vi "test_RT driver Mockup.vi"() -> ()   [LabVIEW 2020]
uses:
  <instrlib>/BTI1553Lib/Public/Controls/1553 RT Transfer Type.ctl
  <instrlib>/BTI1553Lib/Public/Controls/1553 Transfer Direction.ctl
  _typedefs/rtdm_states_type.ctl
  <instrlib>/BTICardLib/Public/Controls/1553 Record.ctl
  _typedefs/rtdm_reference_types.ctl
  <extravilib>/ChannelInstances/Tag-bool/Write With Abort.vi
  <extravilib>/ChannelInstances/Tag-bool/Read With Abort.vi
  <instrlib>/BTICardLib/Private/Initialize By Card Number and Core Number.vi
  <instrlib>/BTI1553Lib/Private/Channel/Configure/Configure All From XML.vi
  <instrlib>/BTI1553Lib/Private/RT/Configure/Get RT Xfer Handle.vi
  <extravilib>/ChannelInstances/Tag-bool/Instantiate.vi
  <extravilib>/ChannelInstances/Tag-bool/Endpoint.vi
  <extravilib>/ChannelInstances/Tag-bool/EndpointRead.vi
  <instrlib>/BTICardLib/BTICardLV.lvlib
  <instrlib>/BTI1553Lib/BTI1553LV.lvlib
  <extravilib>/ChannelInstances/Tag-bool.lvlib
panel:
  out "data word count out":i32
  out "error out async":errorcluster
  out "error out inline":errorcluster
  in  "Stop operating":bool
  in  "Async period ms":u32=10
  in  "data words":u16[](array[numeric]) format="%04x"
  in  "message type":enum16{"BC-RT", "RT-BC_RT"}(ring)
  out "byte count":i32
  out "last record":T1 {"type" format="%04x"; "activity" format="%04x"; "error" format="%04x"; "cwd1" format="%04x"; "cwd2" format="%04x"; "swd1" format="%04x"; "swd2" format="%04x"; "data" format="%04x"}
  in  "inline period mS":u32=10
  out "current state":T2=enum."Close"
  in  "transfer sa number or mc number":i32=2
  in  "transfer direction":T3 items=["DIRECTION_RECEIVE", "DIRECTION_TRANSMIT"]
  in  "transfer type":T4 items=["RTXFER_SUBADDRESS", "RTXFER_MODECODE"]
  in  "rt address":i32=1
  in  "rt channel":i32
  in  "bc command name":string="testTransfer"
  in  "bc channel index":i32
  out "Product String":string="222-555-442"
  out "Card Type":string="OmniBus II cPCIe/PXIe"
  out "channel count out":i32=1
  in  "number of channels":i32=1
  out "XML load time ms":u32=10008
  in  "card number":i32=1
  in  "core number":i32
  in  "configuration file path":path=path "c:/ni-rt/VeriStand/Custom Devices/Ballard - 1553/Board_1__Core_0__.xml"
  out "error out":errorcluster
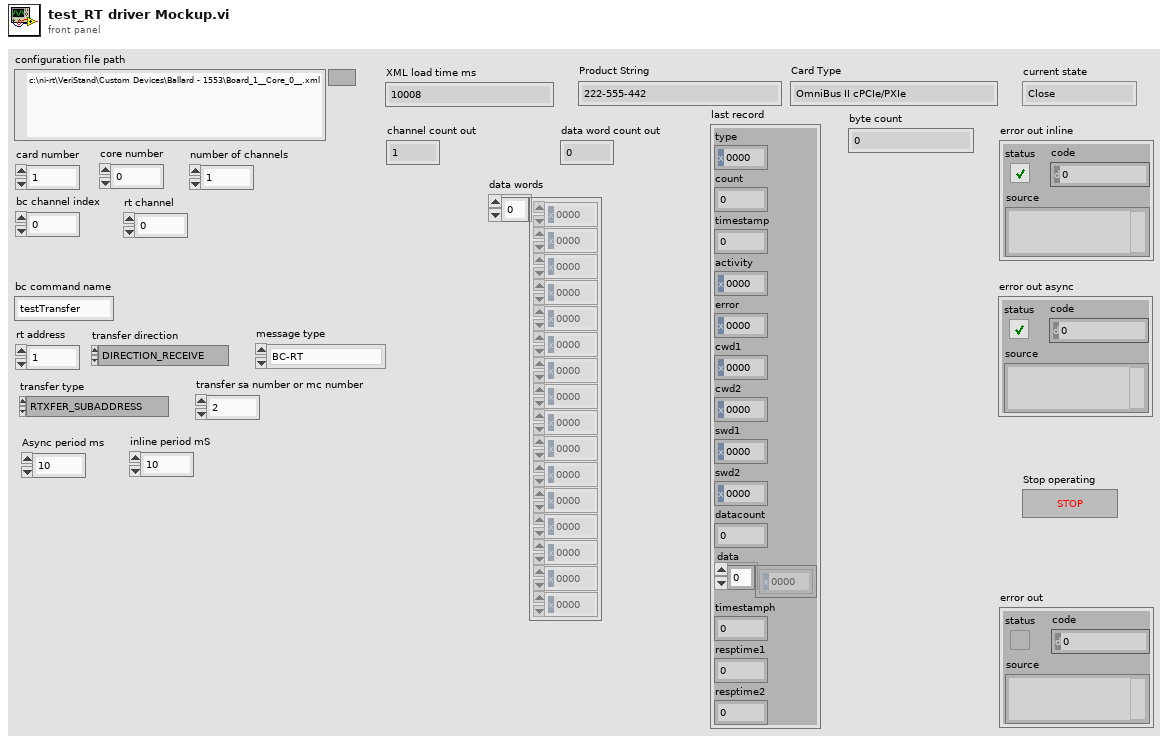
[diagram p1: front panel]
types:
  T1 = typedef "BTICardLV.lvlib/1553 Record.ctl" = cluster{"type":u16, "count":u16, "timestamp":u32, "activity":u16, "error":u16, "cwd1":u16, "cwd2":u16, "swd1":u16, "swd2":u16, "datacount":u16, "data":u16[], "timestamph":u32, "resptime1":u16, "resptime2":u16}
  T2 = typedef "rtdm_states_type.ctl" = enum16{"Initialize", "Get transfer handles", "Operate", "Error", "Close"}
  T3 = typedef "BTI1553LV.lvlib/1553 Transfer Direction.ctl" = u32
  T4 = typedef "BTI1553LV.lvlib/1553 RT Transfer Type.ctl" = u32
  T5 = typedef "rtdm_reference_types.ctl" = cluster{"core handle":u64, "channel handles":u64[], "core reader handle":u64, "bc handle":u64, "bc transfer handle":u64, "rt handle":u64, "rt transfer handle":u64}
  T6 = typedef "Tag-bool.lvlib/))Channel.ctl" = refnum<queue>
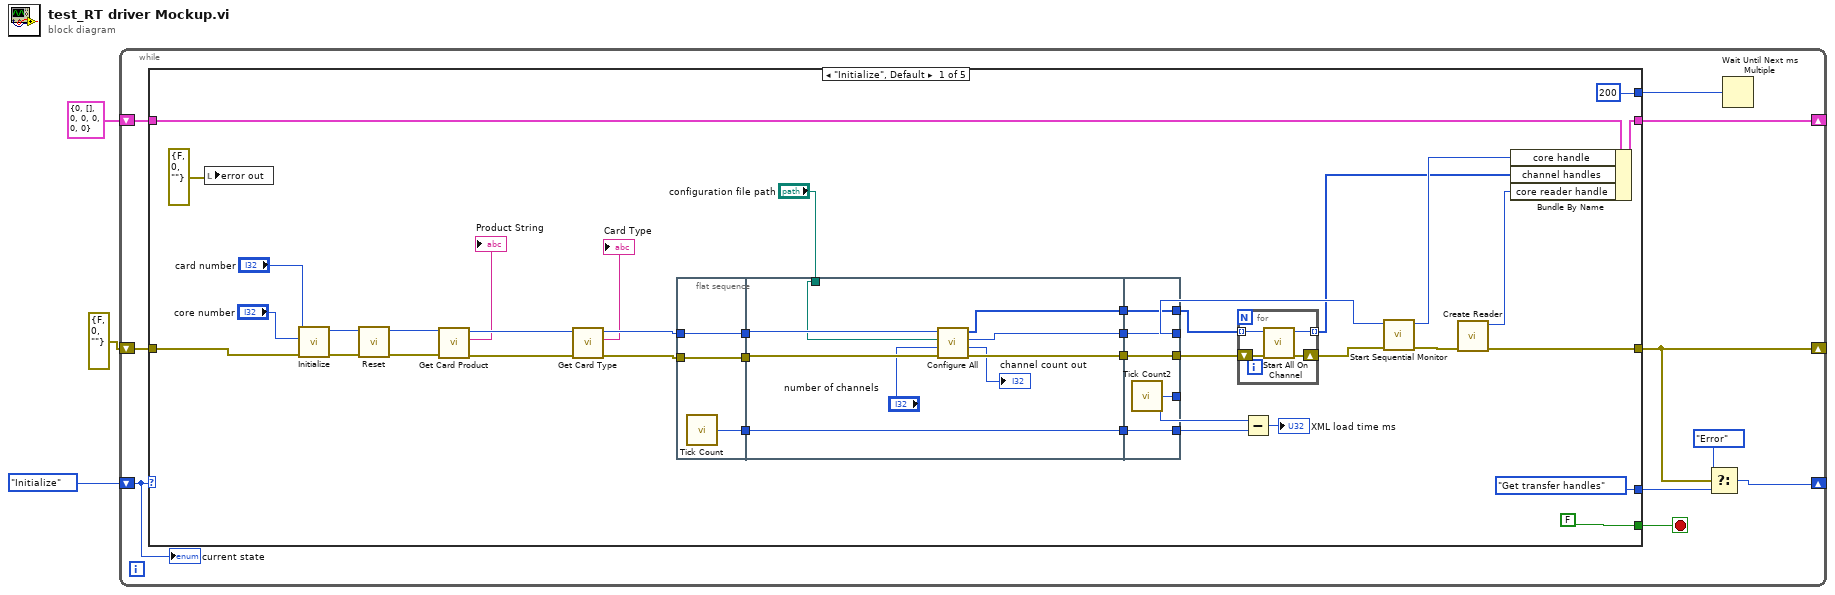
[diagram p0: block diagram]
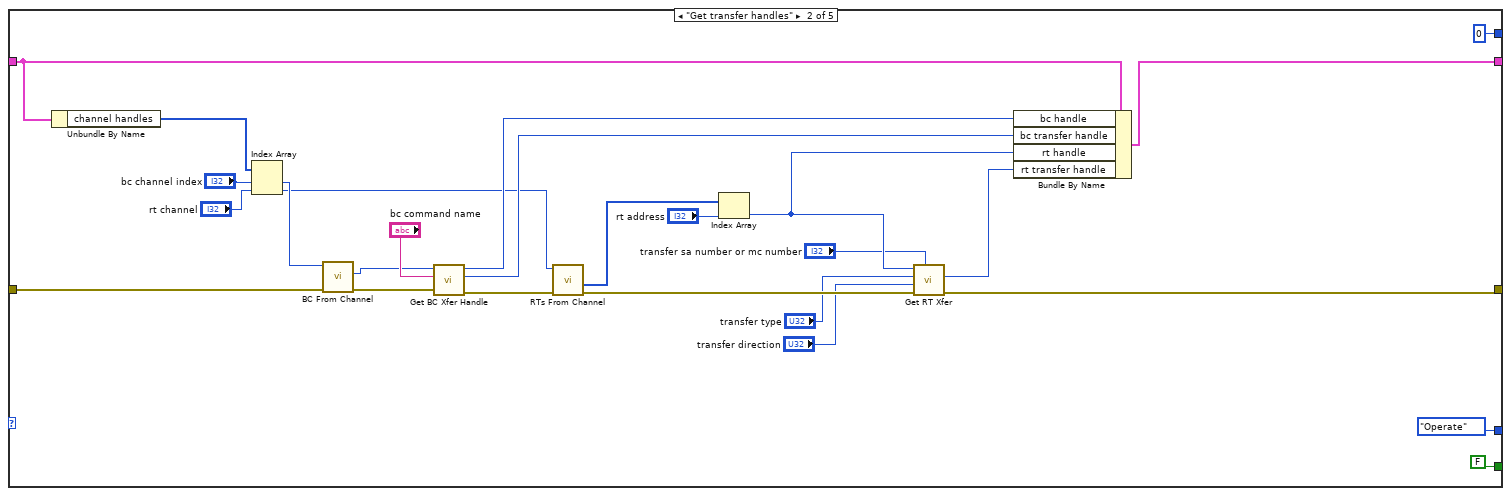
[diagram p2: hidden frame]
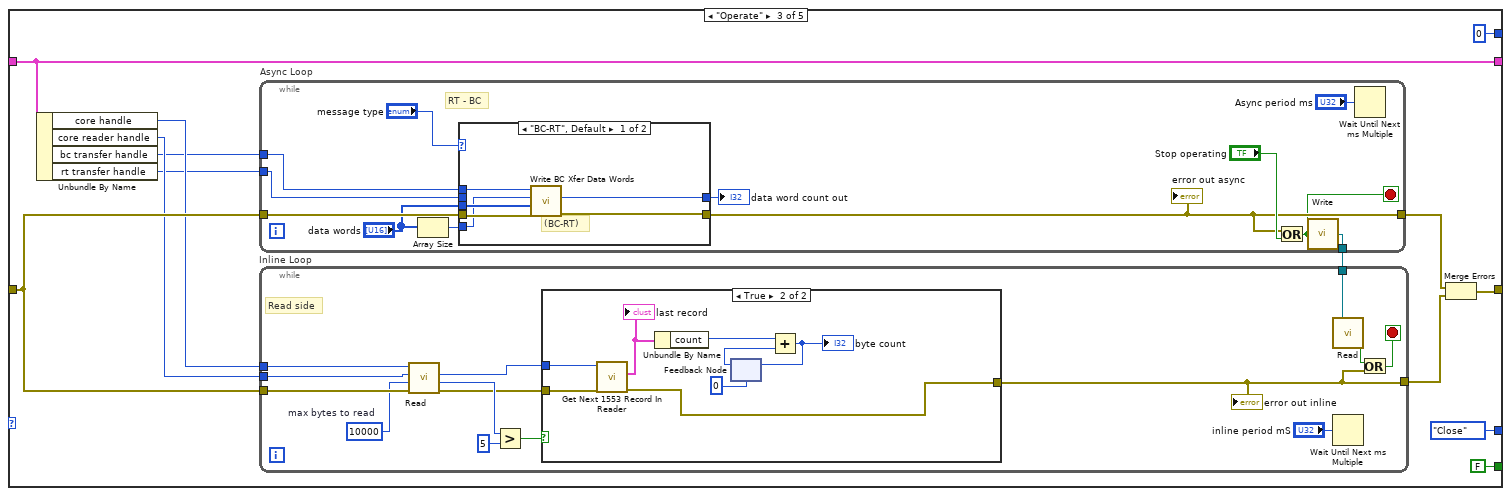
[diagram p3: hidden frame]
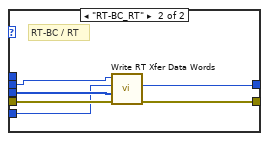
[diagram p4: hidden frame]
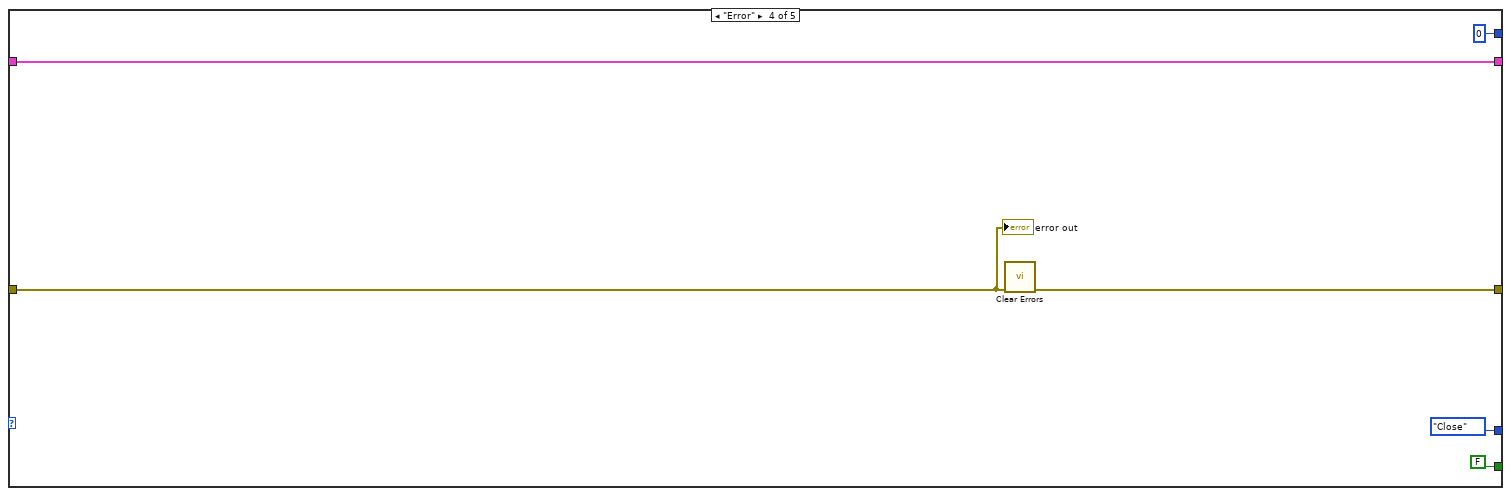
[diagram p6: hidden frame]
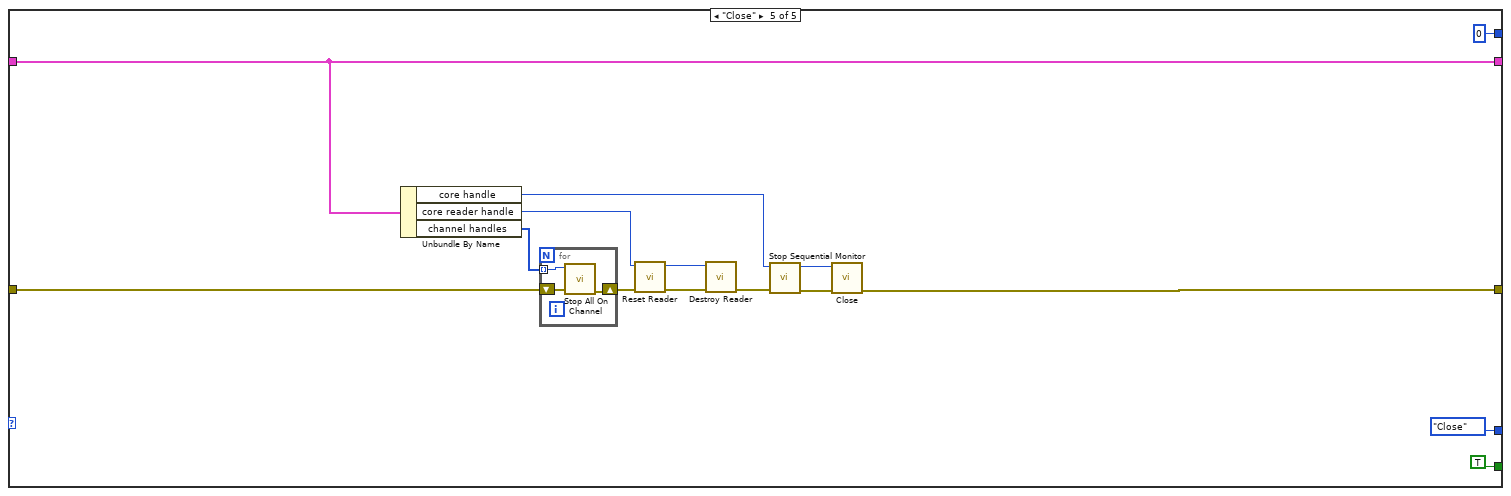
[diagram p7: hidden frame]
diagram:
  n1 = while {
    shift-right: [w8] -> _
    shift-left: rtdm_states_type."Initialize" -> [w13]
    shift-right: [w5] -> _
    shift-left: errorcluster {"status"=FALSE, "code"=0, "source"=""} ("error in (no error)") -> [w9]
    shift-right: [w6] -> _
    shift-left: T5 {"core handle"=0, "channel handles"=[], "core reader handle"=0, "bc handle"=0, "bc transfer handle"=0, "rt handle"=0, "rt transfer handle"=0} -> [w10]
    stop <- w12 stop-if-true
    n2 = case shown="\"Initialize\", Default" w13 {
      tunnel: [FALSE FALSE FALSE FALSE TRUE] -> w12
      tunnel: [u32 200 ("millisecond multiple") u32 0 ("millisecond multiple") u32 0 ("millisecond multiple") u32 0 ("millisecond multiple") u32 0 ("millisecond multiple")] -> w11
      tunnel: w10 -> [w19 w90 w108 w160 w173]
      tunnel: w9 -> [w22 w93 w109 w165 w170]
      tunnel: [w21 w79 w103 w164 w177] -> w5
      tunnel: [rtdm_states_type."Get transfer handles" rtdm_states_type."Operate" rtdm_states_type."Close" rtdm_states_type."Close" rtdm_states_type."Close"] -> w4
      tunnel: [w18 w75 w108 w160 w173] -> w6
      frame "Initialize", Default {
        n3 = local write "error out"(errorcluster {"status"=FALSE, "code"=0, "source"=""} ("error in (no error)")) -> ()
        n4 = call-poly <instrlib>:"Initialize.vi"("error in (no error)"=w22, "core number"="core number", "card number"="card number") -> ("error out"=w23:errorcluster, "core handle out"=w24:u64)  [unwired: 7 in]
        n5 = call <instrlib>:"Reset.vi"("error in (no error)"=w23, "core handle in"=w24) -> ("error out"=w41:errorcluster, "core handle out"=w40:u64)  [unwired: 8 in]
        n6 = call <instrlib>:"Get Card Product.vi"("error in (no error)"=w41, "core handle in"=w40) -> ("error out"=w38:errorcluster, "product string out"=→"Product String":string, "core handle out"=w39:u64)  [unwired: 7 in]
        n7 = call <instrlib>:"Get Card Type.vi"("error in (no error)"=w38, "core handle in"=w39) -> ("error out"=w42:errorcluster, "type string out"=→"Card Type":string, "core handle out"=w43:u64)  [unwired: 7 in]
        n8 = flat-sequence {
          tunnel: w42 -> [w58]
          tunnel: w43 -> [w59]
          tunnel: [w59] -> w50
          tunnel: [w58] -> w49
          tunnel: [w57] -> w48
          tunnel: [w66] -> w47
          tunnel: [w65] -> w46
          tunnel: w50 -> [w68]
          tunnel: w49 -> [w67]
          tunnel: [w64] -> w45
          tunnel: w48 -> [w64]
          tunnel: "configuration file path" -> [w63]
          tunnel: [w62] -> w44
          tunnel: [w72] -> w31
          tunnel: [w73] -> w33
          tunnel: w47 -> [w73]
          tunnel: w46 -> [w72]
          tunnel: [w71] -> w27
          tunnel: [w70] -> w28
          tunnel: w45 -> [w70]
          tunnel: [w69] -> w32
          tunnel: w44 -> [w69]
          frame #0 {
            n9 = call "Tick Count"() -> ("Tick Count(mSec)"=w57:u32)
          }
          frame #1 {
            n10 = call-poly <instrlib>:"Configure All.vi"("error in (no error)"=w67, "channel handle array size in"="number of channels", "configuration file path"=w63, "core handle in"=w68) -> ("error out"=w65:errorcluster, "channel count out"=→"channel count out":i32, "core handle out"=w66:u64, "channel handles out"=w62:u64[])  [unwired: 4 in]
          }
          frame #2 {
            n11 = call "Tick Count2"() -> ("Tick Count(mSec)"=w71:u32)
          }
        }
        n12 = for {
          shift-right: [w55] -> w34
          shift-left: w31 -> [w56]
          tunnel: w32 -> [w54] mode=indexing
          tunnel: [w53] -> w16 mode=indexing
          n13 = call <instrlib>:"Start All On Channel.vi"("error in (no error)"=w56, "channel handle in"=w54) -> ("error out"=w55:errorcluster, "channel handle out"=w53:u64)  [unwired: 8 in]
        }
        n14 = Subtract(x=w27, y=w28) -> (x-y=→"XML load time ms":u32)
        n15 = call <instrlib>:"Start Sequential Monitor.vi"("error in (no error)"=w34, "core handle in"=w33) -> ("error out"=w35:errorcluster, "core handle out"=w17:u64)  [unwired: 8 in]
        n16 = call <instrlib>:"Create Reader.vi"("error in (no error)"=w35) -> ("error out"=w21:errorcluster, "core reader handle out"=w15:u64)  [unwired: 9 in]
        n17 = Bundle By Name(cluster=w19, "core handle"=w17, "channel handles"=w16, "core reader handle"=w15) -> (w18:T5)
      }
      frame "Get transfer handles" {
        n18 = Unbundle By Name(w90) -> ("channel handles"=w92:u64[])
        n19 = Index Array(array=w92, index #1="bc channel index", index #2="rt channel") -> (element #1=w91:u64, element #2=w74:u64)
        n20 = call <instrlib>:"BC From Channel.vi"("error in (no error)"=w93, "channel handle in"=w91) -> ("error out"=w96:errorcluster, "bus controller handle out"=w95:u64)  [unwired: 7 in, 1 out]
        n21 = call <instrlib>:"Get BC Xfer Handle.vi"("error in (no error)"=w96, "bc transfer name"="bc command name", "bus controller handle in"=w95) -> ("error out"=w99:errorcluster, "bc transfer handle out"=w88:u64, "bus controller handle out"=w89:u64)  [unwired: 6 in]
        n22 = call <instrlib>:"RTs From Channel.vi"("error in (no error)"=w99, "channel handle in"=w74) -> ("error out"=w85:errorcluster, "remote terminal handles out"=w87:u64[])  [unwired: 6 in, 2 out]
        n23 = Index Array(array=w87, index="rt address") -> (element=w84:u64)
        n24 = call-poly <instrlib>:"Get RT Xfer.vi"("transfer sa number or mc number"="transfer sa number or mc number", "error in (no error)"=w85, "transfer direction"="transfer direction", "transfer type"="transfer type", "remote terminal handle in"=w84) -> ("error out"=w79:errorcluster, "rt transfer handle out"=w80:u64)  [unwired: 4 in, 1 out]
        n25 = Bundle By Name(cluster=w90, "bc handle"=w89, "bc transfer handle"=w88, "rt handle"=w84, "rt transfer handle"=w80) -> (w75:T5)
      }
      frame "Operate" {
        n26 = Unbundle By Name(w108) -> ("core handle"=w107:u64, "core reader handle"=w106:u64, "bc transfer handle"=w105:u64, "rt transfer handle"=w104:u64)
        n27 = while "Async Loop" {
          tunnel: w109 -> [w124]
          tunnel: w105 -> [w123]
          tunnel: w104 -> [w120]
          tunnel: [w117] -> w102
          tunnel: [w116] -> w100
          stop <- w113 stop-if-true
          # "RT - BC"
          n28 = Array Size(array="data words") -> (size(s)=w114:i32)
          n29 = case shown="\"BC-RT\", Default" "message type" {
            tunnel: w124 -> [w130 w136]
            tunnel: w123 -> [w129 _]
            tunnel: "data words" -> [w128 w134]
            tunnel: w120 -> [_ w135]
            tunnel: [w127 w133] -> w117
            tunnel: [w126 w132] -> w115
            tunnel: w114 -> [w125 w131]
            frame "BC-RT", Default {
              # "(BC-RT)"
              n30 = call <instrlib>:"Write BC Xfer Data Words.vi"("error in (no error)"=w130, "data words"=w128, "data word count in"=w125, "bc transfer handle in"=w129) -> ("error out"=w127:errorcluster, "data word count out"=w126:i32)  [unwired: 5 in, 1 out]
            }
            frame "RT-BC_RT" {
              # "RT-BC / RT"
              n31 = call <instrlib>:"Write RT Xfer Data Words.vi"("error in (no error)"=w136, "data words"=w134, "data word count in"=w131, "rt transfer handle in"=w135) -> ("error out"=w133:errorcluster, "data word count out"=w132:i32)  [unwired: 5 in, 1 out]
            }
          }
          "error out async" <- w117
          "data word count out" <- w115
          n32 = Or(x=w117, y="Stop operating") -> (x .or. y?=w113:bool)
          n33 = call <extravilib>:"Write.vi"("element"=w113) -> ("channel"=w116:T6)  [unwired: 1 out]
          n34 = Wait Until Next ms Multiple(millisecond multiple="Async period ms") -> ()  [unwired: 1 out]
        }
        n35 = while "Inline Loop" {
          tunnel: w109 -> [w149]
          tunnel: w107 -> [w144]
          tunnel: w106 -> [w143]
          tunnel: [w140] -> w101
          tunnel: w100 -> [w139]
          stop <- w137 stop-if-true
          w148 = 10000  # max bytes to read
          # "Read side"
          n36 = call <instrlib>:"Read.vi"("error in (no error)"=w149, "max bytes to read"=w148, "core reader handle in"=w143, "core handle in"=w144) -> ("error out"=w142:errorcluster, "bytes read"=w147:i32, "core reader handle out"=w141:u64)  [unwired: 4 in, 1 out]
          n37 = Greater?(x=w147, y=5) -> (0:w145:bool)
          n38 = case shown="True" w145 {
            tunnel: w142 -> [w151 w159]
            tunnel: w141 -> [_ w158]
            tunnel: [w151 w152] -> w140
            frame False {
            }
            frame True {
              n39 = call <instrlib>:"Get Next 1553 Record In Reader.vi"("error in (no error)"=w159, "core reader handle in"=w158) -> ("error out"=w152:errorcluster, "record out"=w157:T1)  [unwired: 7 in, 1 out]
              "last record" <- w157
              n40 = Unbundle By Name(w157) -> ("count"=w153:u16)
              n41 = feedback #1(0) -> (w154:i32)
              n42 = Add(x=w153, y=w154) -> (x+y=w155:i32)
              "byte count" <- w155
              n43 = feedback-in #1(w155) -> ()
            }
          }
          "error out inline" <- w140
          n44 = call <instrlib>:"Read.vi"("channel"=w139) -> ("element"=w138:bool)  [unwired: 1 in, 1 out]
          n45 = Wait Until Next ms Multiple(millisecond multiple="inline period mS") -> ()  [unwired: 1 out]
          n46 = Or(x=w138, y=w140) -> (x .or. y?=w137:bool)
        }
        n47 = Merge Errors(w102, w101) -> (w103:errorcluster)
      }
      frame "Error" {
        n48 = call <vilib>:"Clear Errors.vi"("error in (no error)"=w165) -> ("error out"=w164:errorcluster)  [unwired: 5 in, 1 out]
        "error out" <- w165
      }
      frame "Close" {
        n49 = Unbundle By Name(w173) -> ("core handle"=w176:u64, "core reader handle"=w168:u64, "channel handles"=w171:u64[])
        n50 = for {
          tunnel: w171 -> [w183] mode=indexing
          shift-right: [w181] -> w169
          shift-left: w170 -> [w182]
          n51 = call <instrlib>:"Stop All On Channel.vi"("error in (no error)"=w182, "channel handle in"=w183) -> ("error out"=w181:errorcluster)  [unwired: 8 in, 1 out]
        }
        n52 = call <instrlib>:"Reset Reader.vi"("error in (no error)"=w169, "reader handle in"=w168) -> ("error out"=w166:errorcluster, "reader handle out"=w167:u64)  [unwired: 8 in]
        n53 = call <instrlib>:"Destroy Reader.vi"("error in (no error)"=w166, "reader handle in"=w167) -> ("error out"=w178:errorcluster)  [unwired: 9 in]
        n54 = call <instrlib>:"Stop Sequential Monitor.vi"("error in (no error)"=w178, "core handle in"=w176) -> ("error out"=w180:errorcluster, "core handle out"=w179:u64)  [unwired: 8 in]
        n55 = call <instrlib>:"Close.vi"("error in (no error)"=w180, "core handle in"=w179) -> ("error out"=w177:errorcluster)  [unwired: 8 in, 1 out]
      }
    }
    n56 = Select(t=rtdm_states_type."Error", s=w5, f=w4) -> (s? t:f=w8:T2)
    n57 = Wait Until Next ms Multiple(millisecond multiple=w11) -> ()  [unwired: 1 out]
    "current state" <- w13
  }
